vi "Whiten.vi"(7 "Opt":enum16{"SVD Method", "Inverse Method"}(ring), 11 "X (Data Matrix)":dbl[][](array[numeric])) -> (0 "Selected":bool[](array[boolean]), 1 "Dewhitening Matrix":dbl[][](array[numeric]), 2 "Whitening Matrix":dbl[][](array[numeric]), 3 "newVector":T1)   [LabVIEW 2014]
uses:
  <vilib>/Analysis/Matrix/Datatypes/RealMatrix.ctl
  <vilib>/Analysis/7linalg.llb/SVD Option.ctl
  <vilib>/Analysis/7linalg.llb/Eigenvalue and Vectors Output Option.ctl
  <vilib>/Analysis/baseanly.llb/Mean (DBL).vi
  <vilib>/Analysis/baseanly.llb/Real A x B.vi
  <vilib>/Analysis/7linalg.llb/Real SVD Decomposition.vi
  <vilib>/Analysis/7linalg.llb/Real Eigenvalues and Vectors.vi
  <vilib>/Analysis/NI_AALPro.lvlib
  <vilib>/gmath/NI_Gmath.lvlib
  <vilib>/Analysis/NI_AALBase.lvlib
  <vilib>/Analysis/Matrix/NI_Matrix.lvlib
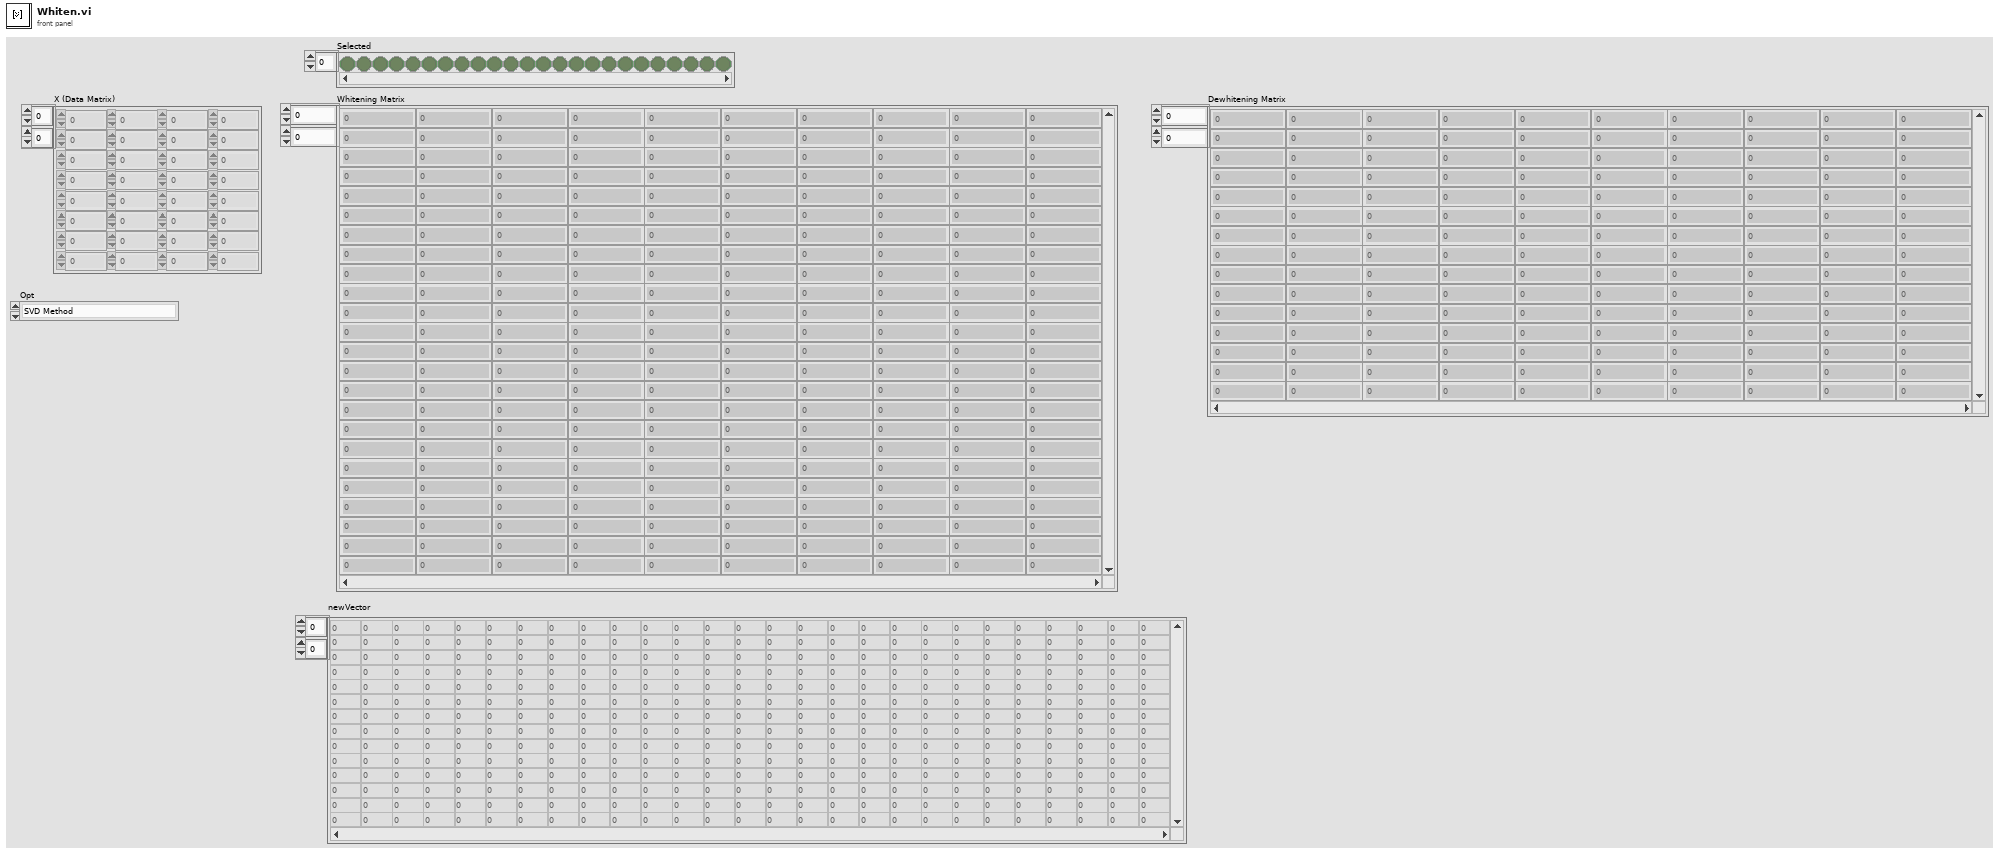
[diagram p1: front panel]
types:
  T1 = typedef "NI_Matrix.lvlib/RealMatrix.ctl" = dbl[][]
  T2 = enum16{"Transpose", "Vertical Flip", "Horizontal Flip", "Rotate 90", "Rotate 180", "Rotate 270", "Diagonal Flip"}
  T3 = typedef "NI_AALPro.lvlib/SVD Option.ctl" = u16
  T4 = typedef "NI_AALPro.lvlib/Eigenvalue and Vectors Output Option.ctl" = i32
  T5 = typedef "NI_Matrix.lvlib/ComplexMatrix.ctl" = cdb[][]
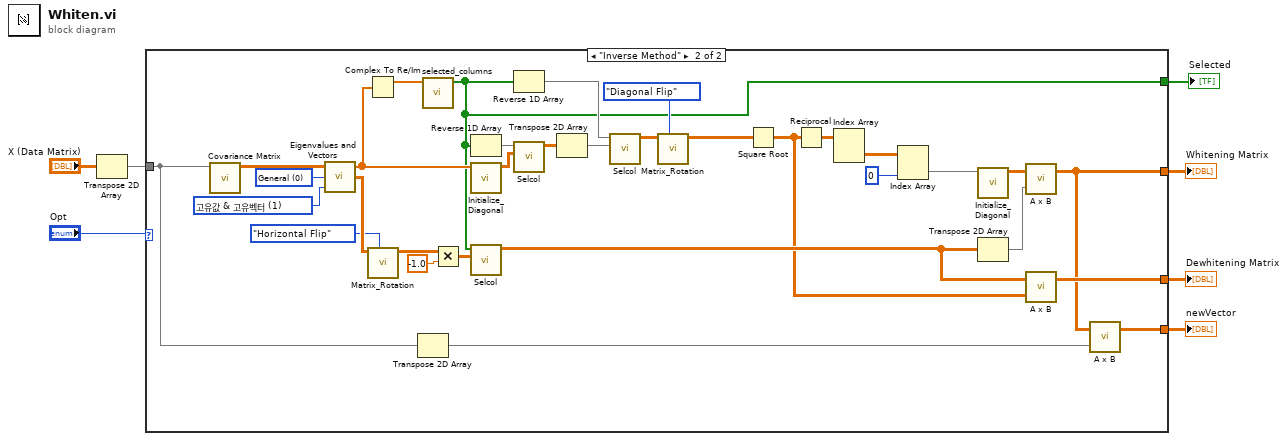
[diagram p0: block diagram]
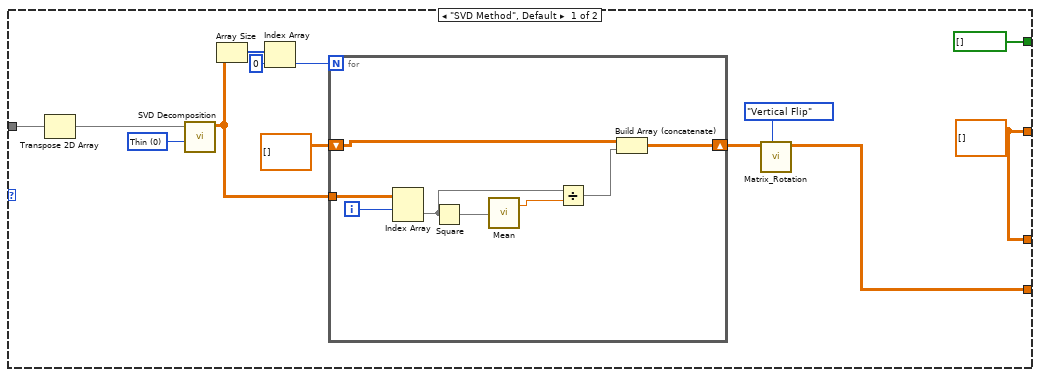
[diagram p2: hidden frame]
diagram:
  n1 = Transpose 2D Array(2D array="X (Data Matrix)") -> (transposed array=w2:dbl[][])
  n2 = case shown="\"Inverse Method\"" "Opt" {
    tunnel: [w13 w36] -> w4
    tunnel: [w13 w35] -> w7
    tunnel: [w9 w33] -> w6
    tunnel: w2 -> [w19 w31]
    tunnel: [bool[] [] w29] -> w1
    frame "SVD Method", Default {
      w13 = T1 [] ("A x B")
      w20 = T3 0 items=["Thin", "Full"] ("SVD option")
      n3 = Transpose 2D Array(2D array=w19) -> (transposed array=w18:dbl[][])
      n4 = call-poly <vilib>:"SVD Decomposition.vi"("SVD option"=w20, "A"=w18) -> ("Matrix U"=w17:T1)  [unwired: 5 in, 4 out]
      n5 = Array Size(array=w17) -> (size(s)=w16:i32[])
      n6 = Index Array(array=w16, index=0) -> (element=w15:i32)
      n7 = for {
        N: w15 -> [_]
        tunnel: w17 -> [w28]
        shift-right: [w22] -> w11
        shift-left: dbl[][] [] -> [w21]
        i -> [w27]
        n8 = Index Array(array=w28, index (row)=w27) -> (element=w24:dbl[])  [unwired: 1 in]
        n9 = Square(x=w24) -> (x^2=w26:dbl[])
        n10 = call-poly <vilib>:"Mean.vi"("X"=w26) -> ("mean"=w25:dbl)  [unwired: 1 out]
        n11 = Divide(x=w24, y=w25) -> (x/y=w23:dbl[])
        n12 = Build Array (concatenate)(w21, w23) -> (w22:dbl[][])
      }
      n13 = call "Matrix_Rotation.vi"("Opt"=T2."Vertical Flip", "Input"=w11) -> ("Output"=w9:dbl[][])  [unwired: 9 in]
    }
    frame "Inverse Method" {
      w54 = 0 items=["General", "Symmetric"] ("matrix type")
      w60 = T4 1 items=["고유값", "고유값 & 고유벡터"] ("output option")
      n14 = call <vilib>:"Covariance Matrix.vi"("X"=w31) -> ("covariance matrix V"=w59:T1)  [unwired: 9 in, 1 out]
      n15 = call-poly <vilib>:"Eigenvalues and Vectors.vi"("output option"=w60, "matrix type"=w54, "Input Matrix"=w59) -> ("Eigenvectors"=w58:T5, "Eigenvalues"=w53:cdb[])  [unwired: 1 out]
      n16 = Complex To Re/Im(x + iy=w53) -> (x=w52:dbl[])  [unwired: 1 out]
      n17 = call "Matrix_Rotation.vi"("Opt"=T2."Horizontal Flip", "Input"=w58) -> ("Output"=w56:dbl[][])  [unwired: 9 in]
      n18 = Transpose 2D Array(2D array=w31) -> (transposed array=w34:dbl[][])
      n19 = call "selected_columns.vi"("eigen value (real)"=w52) -> ("Selected"=w29:bool[])  [unwired: 10 in]
      n20 = Multiply(x=w56, y=-1.0) -> (x*y=w51:dbl[][])
      n21 = Reverse 1D Array(array=w29) -> (reversed array=w49:bool[])
      n22 = call "Initialize_Diagonal.vi"("Eigen Value"=w53) -> ("output matrix"=w50:T1)  [unwired: 10 in]
      n23 = call "Selcol.vi"("Array in"=w51, "Selected"=w29) -> ("Array out"=w39:dbl[][])  [unwired: 9 in]
      n24 = Reverse 1D Array(array=w29) -> (reversed array=w30:bool[])
      n25 = call "Selcol.vi"("Array in"=w50, "Selected"=w49) -> ("Array out"=w48:dbl[][])  [unwired: 9 in]
      n26 = Transpose 2D Array(2D array=w48) -> (transposed array=w40:dbl[][])
      n27 = call "Selcol.vi"("Array in"=w40, "Selected"=w30) -> ("Array out"=w41:dbl[][])  [unwired: 9 in]
      n28 = call "Matrix_Rotation.vi"("Opt"=T2."Diagonal Flip", "Input"=w41) -> ("Output"=w38:dbl[][])  [unwired: 9 in]
      n29 = Square Root(x=w38) -> (sqrt(x)=w37:dbl[][])
      n30 = Reciprocal(x=w37) -> (1/x=w47:dbl[][])
      n31 = Index Array(array=w47) -> (element=w46:dbl[][])  [unwired: 2 in]
      n32 = Index Array(array=w46, index (col)=0 ("index (row)")) -> (element=w45:dbl[])  [unwired: 1 in]
      n33 = call "Initialize_Diagonal.vi"("Eigen Value"=w45) -> ("output matrix"=w32:T1)  [unwired: 10 in]
      n34 = Transpose 2D Array(2D array=w39) -> (transposed array=w43:dbl[][])
      n35 = call-poly <vilib>:"A x B.vi"("B"=w43, "A"=w32) -> ("A x B"=w35:T1)  [unwired: 1 out]
      n36 = call-poly <vilib>:"A x B.vi"("B"=w37, "A"=w39) -> ("A x B"=w36:T1)  [unwired: 1 out]
      n37 = call-poly <vilib>:"A x B.vi"("B"=w34, "A"=w35) -> ("A x B"=w33:T1)  [unwired: 1 out]
    }
  }
  "Whitening Matrix" <- w7
  "newVector" <- w6
  "Dewhitening Matrix" <- w4
  "Selected" <- w1
